vi "Run Banana Test Suite.vi"() -> ()   [LabVIEW 2021]
uses:
  <vilib>/addons/_JKI Toolkits/Caraya/classes/Test Result/Node Results (Extended).ctl
  <vilib>/addons/_JKI Toolkits/Caraya/classes/Test Result/Test Node (Extended).ctl
  <vilib>/addons/_JKI Toolkits/Caraya/classes/Test Result/Test Registration Data.ctl
  <vilib>/addons/_JKI Toolkits/Caraya/classes/Test Result/Assert Event Data (Extended).ctl
  Banana.Caraya/Platano.CarayaTestSuite/Platano.CarayaTestSuite.lvclass
  C:/Repositories/LVOS/Bananas/lv-src/Bananas/Platano/Platano.lvclass
  <vilib>/addons/_JKI Toolkits/Caraya/classes/Test Result/Test Result.lvclass
  Bananas/Platano/Platano.lvclass
  Bananas/Bananas.lvlib
panel:
  out "Config Map":map{string, string}(c390)
  out "Test Results":T1[](array[typedef])
  in  "error in":errorcluster
  out "error out":errorcluster
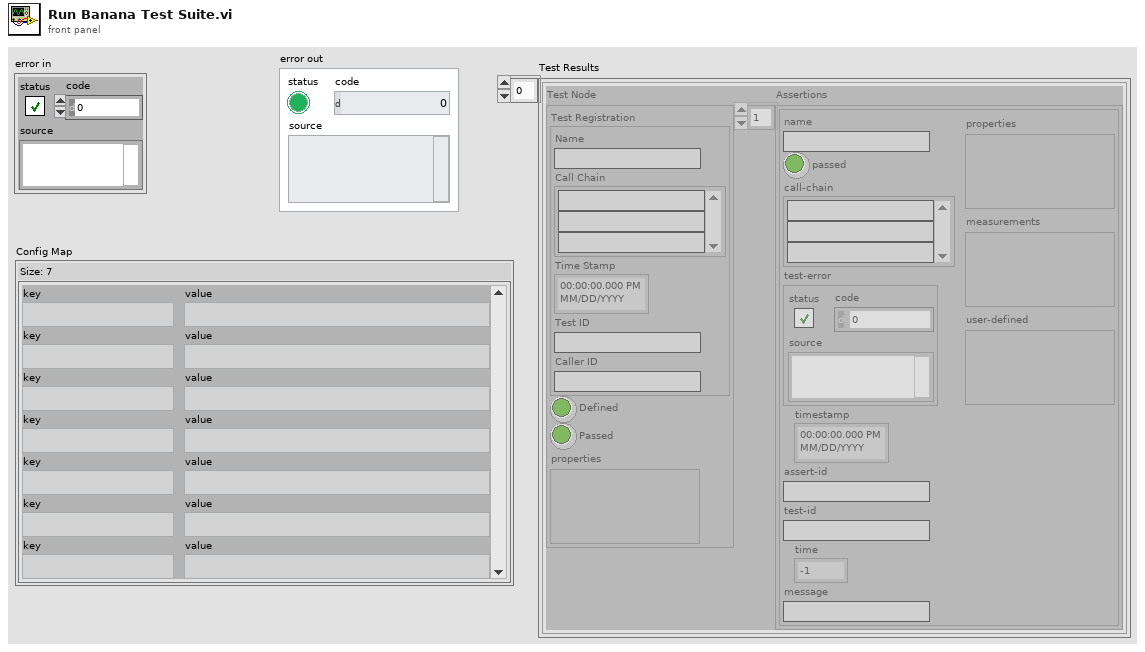
[diagram p1: front panel]
types:
  T1 = typedef "Caraya.lvlib/Test Result.lvclass/Node Results (Extended).ctl" = cluster{"Test Node":T2, "Assertions":T4[]}
  T2 = typedef "Caraya.lvlib/Test Result.lvclass/Test Node (Extended).ctl" = cluster{"Test Registration":T3, "Defined":bool, "Passed":bool, "properties":variant}
  T3 = typedef "Caraya.lvlib/Test Result.lvclass/Test Registration Data.ctl" = cluster{"Name":string, "Call Chain":string[], "Time Stamp":timestamp, "Test ID":string, "Caller ID":string}
  T4 = typedef "Caraya.lvlib/Test Result.lvclass/Assert Event Data (Extended).ctl" = cluster{"name":string, "passed":bool, "call-chain":string[], "test-error":errorcluster, "timestamp":timestamp, "assert-id":string, "test-id":string, "time":dbl, "message":string, "properties":variant, "measurements":variant, "user-defined":variant}
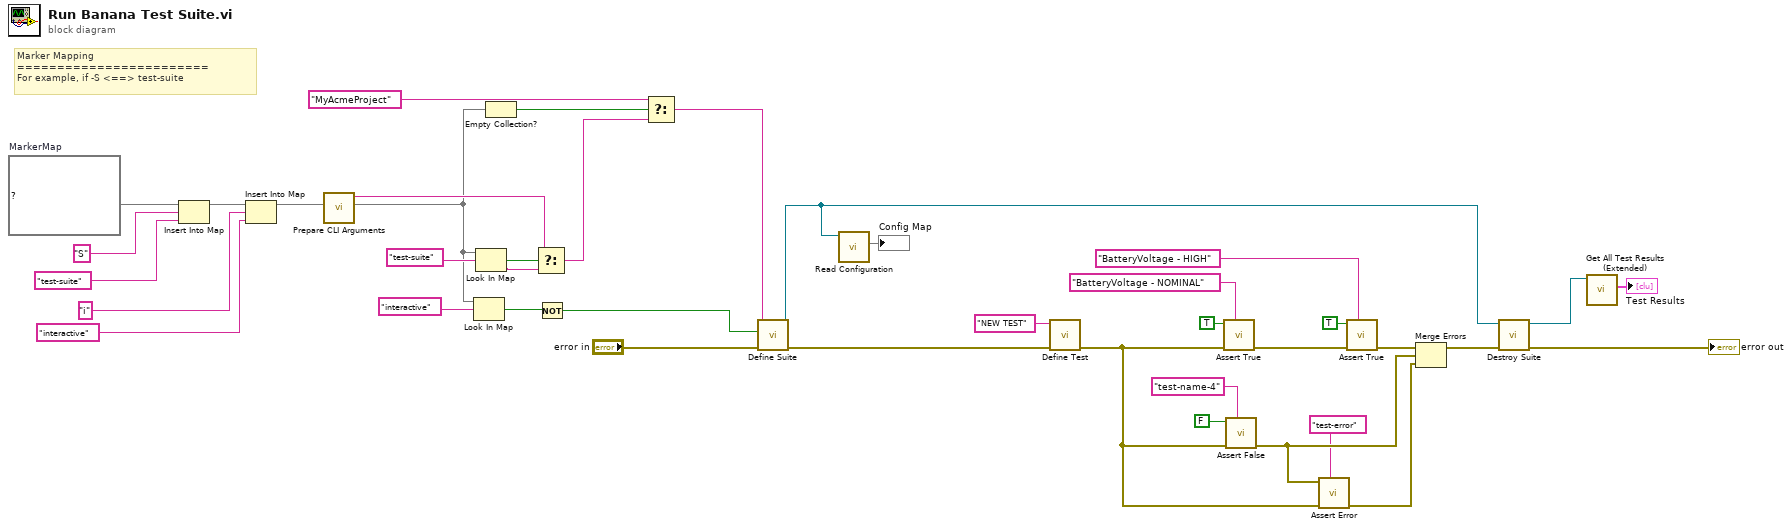
[diagram p0: block diagram]
diagram:
  w19 = map{string, string} {}  # MarkerMap
  # "Marker Mapping\n========================\nFor example, if -S <==> test-suite"
  n1 = Insert Into Map(map in=w19, key="S" ("element"), value="test-suite" ("element")) -> (map out=w11:map{string, string})  [unwired: 2 out]
  n2 = Insert Into Map(map in=w11, key="i" ("element"), value="interactive" ("element")) -> (map out=w10:map{string, string})  [unwired: 2 out]
  n3 = call "Prepare CLI Arguments.vi"("Marker Mapping"=w10) -> ("Arguments"=w4:map{string, string}, "application name"=w14:string)  [unwired: 8 in, 1 out]
  n4 = Look In Map(map=w4, key="interactive" ("element")) -> (key not found?=w7:bool)  [unwired: 1 in, 1 out]
  n5 = Look In Map(map=w4, key="test-suite" ("element")) -> (key not found?=w15:bool, value=w13:string)  [unwired: 1 in]
  n6 = Empty Collection?(1:w4) -> (0:w3:bool)
  n7 = Select(t=w14, s=w15, f=w13) -> (s? t:f=w2:string)
  n8 = Not(x=w7) -> (.not. x?=w6:bool)
  n9 = Select(t="MyAcmeProject" ("element"), s=w3, f=w2) -> (s? t:f=w1:string)
  n10 = call "Define Suite.vi"("error in"="error in", "Interactive"=w6, "Label (VI Title)"=w1) -> ("error out"=w25:errorcluster, "Platano"=w21:refnum<class "Platano.CarayaTestSuite.lvclass">)  [unwired: 6 in, 1 out]
  n11 = call "Read Configuration.vi"("Platano in"=w21) -> ("Config Map"=→"Config Map":map{string, string})  [unwired: 8 in, 2 out]
  n12 = call "Define Test.vi"("error in"=w25, "Label (VI Title)"="NEW TEST") -> ("error out"=w28:errorcluster)  [unwired: 8 in, 1 out]
  n13 = call "Assert True.vi"("Label"="BatteryVoltage - NOMINAL", "error in"=w28, "True?"=TRUE) -> ("error out"=w36:errorcluster)  [unwired: 7 in, 1 out]
  n14 = call "Assert False.vi"("Label"="test-name-4", "error in"=w28, "False?"=FALSE ("True?")) -> ("error out"=w30:errorcluster)  [unwired: 7 in, 1 out]
  n15 = call "Assert Error.vi"("Label"="test-error", "error in"=w28, "error"=w30) -> ("error out"=w27:errorcluster)  [unwired: 7 in, 1 out]
  n16 = call "Assert True.vi"("Label"="BatteryVoltage - HIGH", "error in"=w36, "True?"=TRUE) -> ("error out"=w35:errorcluster)  [unwired: 7 in, 1 out]
  n17 = Merge Errors(w35, w30, w27) -> (w24:errorcluster)
  n18 = call "Destroy Suite.vi"("error in"=w24, "Platano"=w21) -> ("error out"=→"error out":errorcluster, "Test Suite Results"=w23:refnum<class "Test Result.lvclass">)  [unwired: 8 in]
  n19 = call <vilib>:"Get All Test Results (Extended).vi"("Test Result in"=w23) -> ("Test Results"=→"Test Results":T1[])  [unwired: 8 in, 2 out]
